vi "Get_All_Info_DAQmx_Task.vi"(11 "task":refnum<k21>) -> ()   [LabVIEW 2016]
uses:
  <resource>/objmgr/daqmx.rc
panel:
  out "UpdateVersion":u32
  out "MinorVersion":u32
  out "MajorVersion":u32
  out "DevNames":tag[](array[tag])
  out "error out":errorcluster
  in  "error in (no error)":errorcluster
  out "output cluster":T1
  out "MNK":T2(array[cluster])=[{"Channels"=["PXI1Slot2/ai0", "PXI1Slot2/ai1"], "DeviceIsSimulated"=[FALSE], "ProductCategory"=[14649], "ProductType"=["PXI-4461"], "ProductNum"=[29299], "DevSerialNum"=[20525895], "Accessory.ProductTypes"=[[""]], "Accessory.ProductNums"=[[0]], "Accessory.SerialNums"=[[0]], "CarrierSerialNum"=[0], "Name"="", "NumChans"=2, "NumDevices"=1, "Done"=FALSE}, {"Channels"=["PXI1Slot3/ai0", "PXI1Slot3/ai1"], "DeviceIsSimulated"=[FALSE], "ProductCategory"=[14649], "ProductType"=["PXI-4461"], "ProductNum"=[29299], "DevSerialNum"=[21344870], "Accessory.ProductTypes"=[[""]], "Accessory.ProductNums"=[[0]], "Accessory.SerialNums"=[[0]], "CarrierSerialNum"=[0], "Name"="", "NumChans"=2, "NumDevices"=1, "Done"=FALSE}, {"Channels"=["PXI1Slot5/ai0", "PXI1Slot5/ai1"], "DeviceIsSimulated"=[FALSE], "ProductCategory"=[14649], "ProductType"=["PXI-4461"], "ProductNum"=[29299], "DevSerialNum"=[20763706], "Accessory.ProductTypes"=[[""]], "Accessory.ProductNums"=[[0]], "Accessory.SerialNums"=[[0]], "CarrierSerialNum"=[0], "Name"="", "NumChans"=2, "NumDevices"=1, "Done"=FALSE}, {"Channels"=["PXI1Slot7/ai0", "PXI1Slot7/ai1"], "DeviceIsSimulated"=[FALSE], "ProductCategory"=[14649], "ProductType"=["PXI-4461"], "ProductNum"=[10400], "DevSerialNum"=[14550922], "Accessory.ProductTypes"=[[""]], "Accessory.ProductNums"=[[0]], "Accessory.SerialNums"=[[0]], "CarrierSerialNum"=[0], "Name"="", "NumChans"=2, "NumDevices"=1, "Done"=FALSE}, {"Channels"=["PXI1Slot2/ao0", "PXI1Slot2/ao1"], "DeviceIsSimulated"=[FALSE], "ProductCategory"=[14649], "ProductType"=["PXI-4461"], "ProductNum"=[29299], "DevSerialNum"=[20525895], "Accessory.ProductTypes"=[[""]], "Accessory.ProductNums"=[[0]], "Accessory.SerialNums"=[[0]], "CarrierSerialNum"=[0], "Name"="", "NumChans"=2, "NumDevices"=1, "Done"=FALSE}, {"Channels"=["PXI1Slot3/ao0", "PXI1Slot3/ao1"], "DeviceIsSimulated"=[FALSE], "ProductCategory"=[14649], "ProductType"=["PXI-4461"], "ProductNum"=[29299], "DevSerialNum"=[21344870], "Accessory.ProductTypes"=[[""]], "Accessory.ProductNums"=[[0]], "Accessory.SerialNums"=[[0]], "CarrierSerialNum"=[0], "Name"="", "NumChans"=2, "NumDevices"=1, "Done"=FALSE}, {"Channels"=["PXI1Slot5/ao0", "PXI1Slot5/ao1"], "DeviceIsSimulated"=[FALSE], "ProductCategory"=[14649], "ProductType"=["PXI-4461"], "ProductNum"=[29299], "DevSerialNum"=[20763706], "Accessory.ProductTypes"=[[""]], "Accessory.ProductNums"=[[0]], "Accessory.SerialNums"=[[0]], "CarrierSerialNum"=[0], "Name"="", "NumChans"=2, "NumDevices"=1, "Done"=FALSE}, {"Channels"=["PXI1Slot7/ao0", "PXI1Slot7/ao1"], "DeviceIsSimulated"=[FALSE], "ProductCategory"=[14649], "ProductType"=["PXI-4461"], "ProductNum"=[10400], "DevSerialNum"=[14550922], "Accessory.ProductTypes"=[[""]], "Accessory.ProductNums"=[[0]], "Accessory.SerialNums"=[[0]], "CarrierSerialNum"=[0], "Name"="", "NumChans"=2, "NumDevices"=1, "Done"=FALSE}]
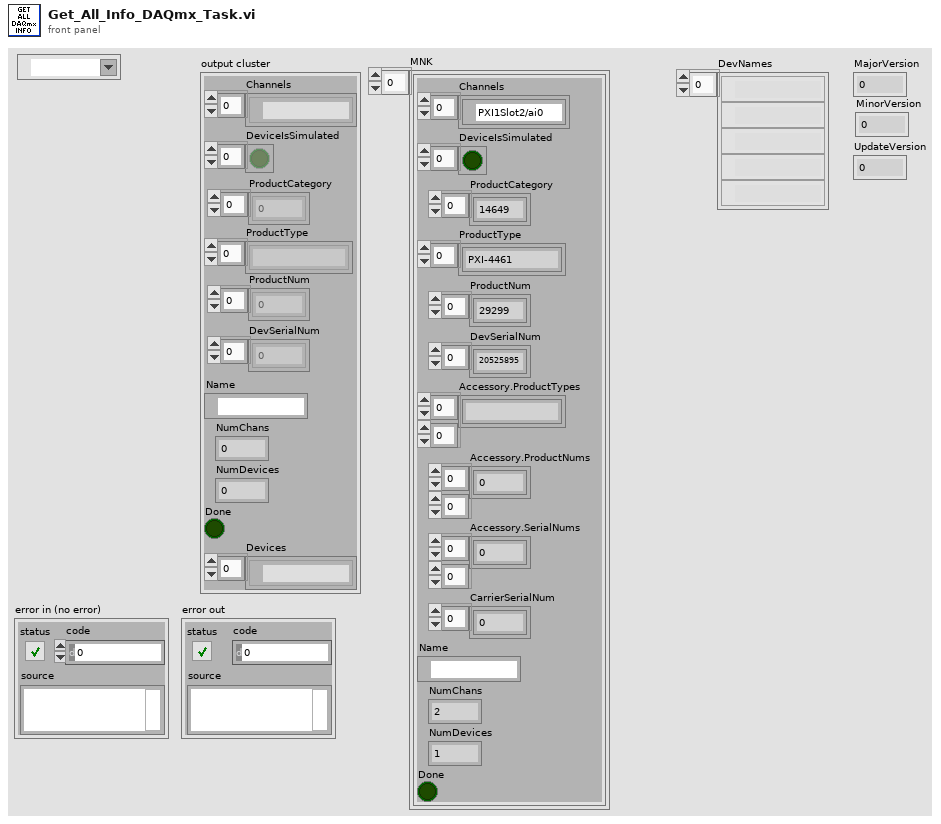
[diagram p1: front panel]
types:
  T1 = cluster{"Channels":refnum<k21>[], "DeviceIsSimulated":bool[], "ProductCategory":i32[], "ProductType":string[], "ProductNum":u32[], "DevSerialNum":u32[], "Name":refnum<k21>, "NumChans":u32, "NumDevices":u32, "Done":bool, "Devices":tag[]}
  T2 = cluster{"Channels":refnum<k21>[], "DeviceIsSimulated":bool[], "ProductCategory":i32[], "ProductType":string[], "ProductNum":u32[], "DevSerialNum":u32[], "Accessory.ProductTypes":string[][], "Accessory.ProductNums":u32[][], "Accessory.SerialNums":u32[][], "CarrierSerialNum":u32[], "Name":refnum<k21>, "NumChans":u32, "NumDevices":u32, "Done":bool}[]
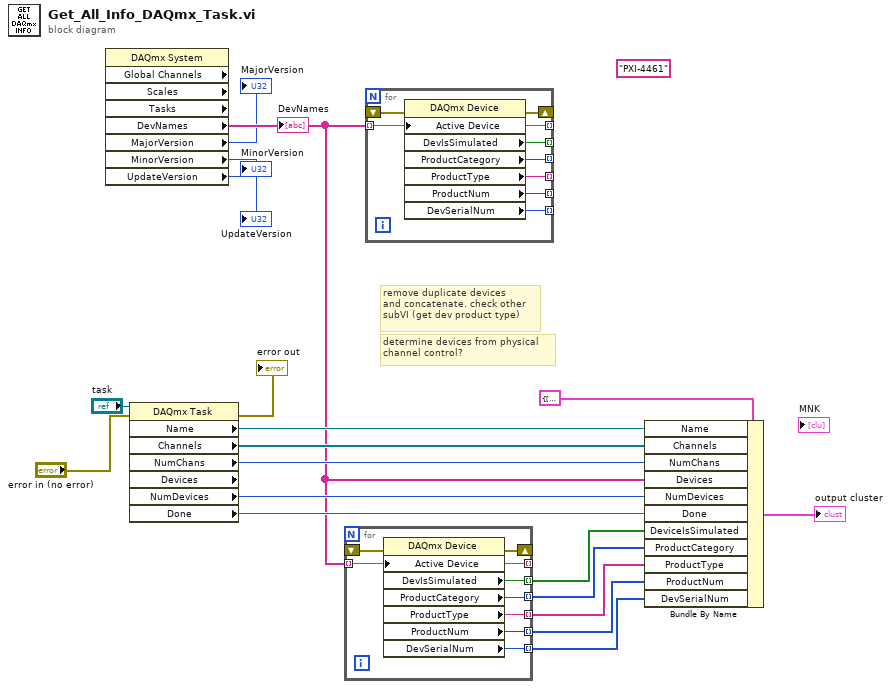
[diagram p0: block diagram]
diagram:
  (unwired) "PXI-4461" ("ProductType")
  # "determine devices from physical\nchannel control?"
  # "remove duplicate devices\nand concatenate. check other\nsubVI (get dev product type)"
  n1 = property class="DAQmx System" props=["Global Channels", "Scales", "Tasks", "DevNames", "MajorVersion", "MinorVersion", "UpdateVersion"]() -> ("DevNames"=w5:tag[], "MajorVersion"=→"MajorVersion":u32, "MinorVersion"=→"MinorVersion":u32, "UpdateVersion"=→"UpdateVersion":u32)  [unwired: 2 in, 5 out]
  "DevNames" <- w5
  n2 = property class="DAQmx Task" props=["Name", "Channels", "NumChans", "Devices", "NumDevices", "Done"](reference="task", error in="error in (no error)") -> (error out=→"error out":errorcluster, "Name"=w19:refnum<k21>, "Channels"=w18:refnum<k21>[], "NumChans"=w17:u32, "NumDevices"=w7:u32, "Done"=w16:bool)  [unwired: 2 out]
  n3 = for {
    tunnel: w5 -> [w22] mode=indexing
    tunnel: [w27] -> w15 mode=indexing
    tunnel: [w26] -> w14 mode=indexing
    tunnel: [w25] -> w13 mode=indexing
    tunnel: [w24] -> w12 mode=indexing
    tunnel: [w23] -> w11 mode=indexing
    tunnel: [w22] -> _ mode=indexing
    shift-right: [w21] -> _
    shift-left: _ -> [w20]
    n4 = property class="DAQmx Device"(error in=w20, "Active Device"=w22) -> (error out=w21:errorcluster, "DevIsSimulated"=w27:bool, "ProductCategory"=w26:i32, "ProductType"=w25:string, "ProductNum"=w24:u32, "DevSerialNum"=w23:u32)  [unwired: 1 in, 1 out]
  }
  n5 = for {
    tunnel: w5 -> [w30] mode=indexing
    tunnel: [w35] -> _ mode=indexing
    tunnel: [w34] -> _ mode=indexing
    tunnel: [w33] -> _ mode=indexing
    tunnel: [w32] -> _ mode=indexing
    tunnel: [w31] -> _ mode=indexing
    tunnel: [w30] -> _ mode=indexing
    shift-right: [w29] -> _
    shift-left: _ -> [w28]
    n6 = property class="DAQmx Device"(error in=w28, "Active Device"=w30) -> (error out=w29:errorcluster, "DevIsSimulated"=w35:bool, "ProductCategory"=w34:i32, "ProductType"=w33:string, "ProductNum"=w32:u32, "DevSerialNum"=w31:u32)  [unwired: 1 in, 1 out]
  }
  n7 = Bundle By Name(cluster=T1 {"Channels"=[], "DeviceIsSimulated"=[], "ProductCategory"=[], "ProductType"=[], "ProductNum"=[], "DevSerialNum"=[], "Name"="", "NumChans"=0, "NumDevices"=0, "Done"=FALSE, "Devices"=[]}, "Name"=w19, "Channels"=w18, "NumChans"=w17, "Devices"=w5, "NumDevices"=w7, "Done"=w16, "DeviceIsSimulated"=w15, "ProductCategory"=w14, "ProductType"=w13, "ProductNum"=w12, "DevSerialNum"=w11) -> (→"output cluster":T1)
